vi "HIOKI PW3390 Conf Measure Item sub4.vi"(1 "Power":T1) -> (0 "Power out":bool[][](array[boolean]))   [LabVIEW 2009]
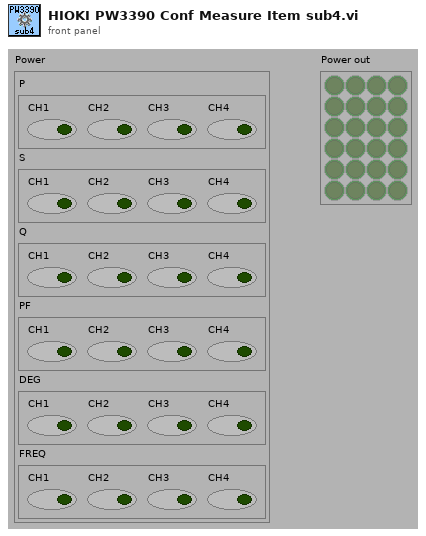
[diagram p1: front panel]
types:
  T1 = cluster{"P":cluster{"CH1":bool, "CH2":bool, "CH3":bool, "CH4":bool}, "S":cluster{"CH1":bool, "CH2":bool, "CH3":bool, "CH4":bool}, "Q":cluster{"CH1":bool, "CH2":bool, "CH3":bool, "CH4":bool}, "PF":cluster{"CH1":bool, "CH2":bool, "CH3":bool, "CH4":bool}, "DEG":cluster{"CH1":bool, "CH2":bool, "CH3":bool, "CH4":bool}, "FREQ":cluster{"CH1":bool, "CH2":bool, "CH3":bool, "CH4":bool}}
  T2 = cluster{"CH1":bool, "CH2":bool, "CH3":bool, "CH4":bool}
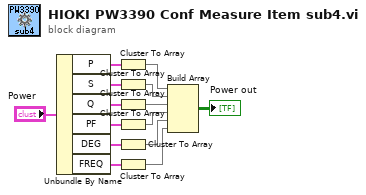
[diagram p0: block diagram]
diagram:
  n1 = Unbundle By Name("Power") -> ("P"=w2:T2, "S"=w3:T2, "Q"=w4:T2, "PF"=w5:T2, "DEG"=w6:T2, "FREQ"=w7:T2)
  n2 = Cluster To Array(cluster=w2) -> (array=w8:bool[])
  n3 = Cluster To Array(cluster=w3) -> (array=w9:bool[])
  n4 = Cluster To Array(cluster=w4) -> (array=w10:bool[])
  n5 = Cluster To Array(cluster=w5) -> (array=w11:bool[])
  n6 = Cluster To Array(cluster=w6) -> (array=w12:bool[])
  n7 = Cluster To Array(cluster=w7) -> (array=w13:bool[])
  n8 = Build Array(w8, w9, w10, w11, w12, w13) -> (→"Power out":bool[][])
